vi "Call Subpanel VI.vi"(8 "error in (no error)":errorcluster, 10 "VI Refnum":refnum<vi>, 11 "CCD Configuration in":refnum<class "CCD Configuration.lvclass">) -> (0 "error out":errorcluster, 3 "CCD Configuration out":refnum<class "CCD Configuration.lvclass">)   [LabVIEW 2016, in "CCD.lvlib" / "CCD Configuration.lvclass"]
uses:
  <userlib>/Common Components/Hardware/CCD/CCD Configuration.lvclass
  <userlib>/Configuration Dialog Actor/Configuration.lvclass
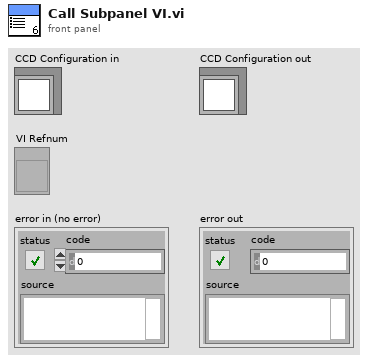
[diagram p1: front panel]
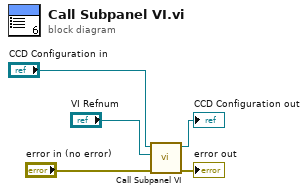
[diagram p0: block diagram]
diagram:
  n1 = call-parent "Call Subpanel VI.vi"("error in (no error)"="error in (no error)", "VI Refnum"="VI Refnum", "Configuration in"="CCD Configuration in") -> ("error out"=→"error out":errorcluster, "Configuration out"=→"CCD Configuration out":refnum<class "CCD Configuration.lvclass">)  [unwired: 7 in]
